vi "Get Alg Result.vi"(8 "error in (no error)":errorcluster, 10 "Alg result":bool=TRUE, 11 "GUI in":refnum<class "GUI.lvclass">) -> (0 "error out":errorcluster, 3 "GUI out":refnum<class "GUI.lvclass">)   [LabVIEW 2020, in "GUI.lvlib" / "GUI.lvclass"]
uses:
  GUI.lvclass
  GUI.lvclass/GUI.ctl
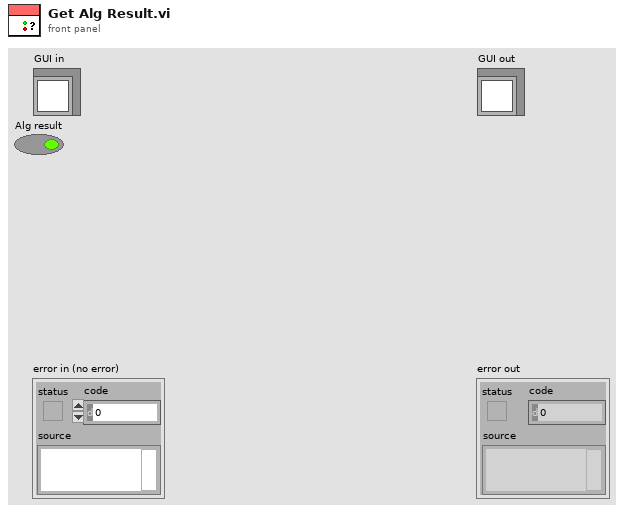
[diagram p1: front panel]
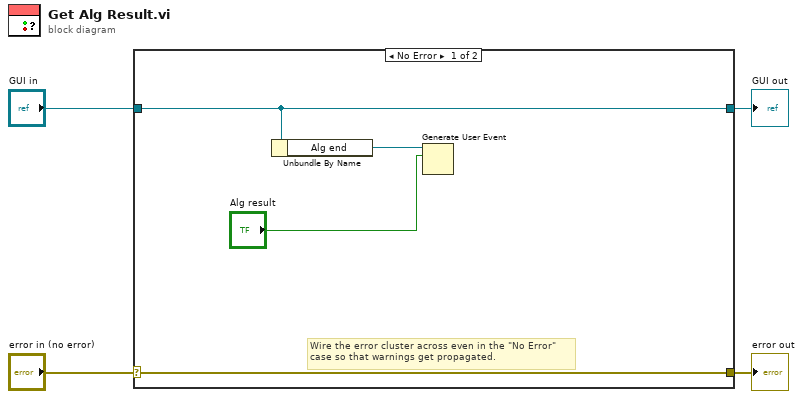
[diagram p0: block diagram]
diagram:
  n1 = case shown="No Error" "error in (no error)" {
    selector: "error in (no error)" -> [w8 w10]
    tunnel: [w8 w10] -> w3
    tunnel: [w7 w9] -> w1
    tunnel: "GUI in" -> [w7 w9]
    frame No Error {
      # "Wire the error cluster across even in the \"No Error\"\ncase so that warnings get propagated."
      n2 = Unbundle By Name(w7) -> ("Alg end"=w6:refnum<user-event>)
      n3 = Generate User Event(user event=w6, event data cluster="Alg result") -> ()  [unwired: 2 in, 2 out]
    }
    frame Error {
    }
  }
  "error out" <- w3
  "GUI out" <- w1
